vi "Get Service Class Instances.vi"() -> (3 "service instances":refnum<class "ServiceBase.lvclass">[](array[class]))   [LabVIEW 2025, in "bus_monitor_server.lvlib"]
uses:
  bus_monitor_server.lvlib
  <vilib>/gRPC/LabVIEW gRPC Servicer/ServiceBase/ServiceBase.lvclass
  RPC Service/Bus_Monitor_API/Bus_Monitor_API.lvclass
  C:/Program Files/National Instruments/LabVIEW 2025/vi.lib/gRPC/LabVIEW gRPC Servicer/ServiceBase/ServiceBase.lvclass
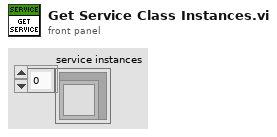
[diagram p1: front panel]
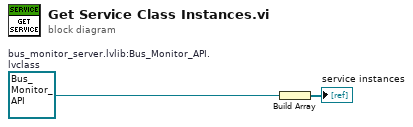
[diagram p0: block diagram]
diagram:
  w1 = refnum<class "Bus_Monitor_API.lvclass"> refnum  # bus_monitor_server.lvlib:Bus_Monitor_API.lvclass
  n1 = Build Array(w1) -> (→"service instances":refnum<class "Bus_Monitor_API.lvclass">[])
